vi "Finalize.vi"(8 "error in (no error)":errorcluster, 11 "Plugin in":refnum<class "Sift TDMS Uploader.lvclass">) -> (0 "error out":errorcluster, 3 "Plugin out":refnum<class "Sift TDMS Uploader.lvclass">)   [LabVIEW 2024, in "Sift TDMS Uploader.lvlib" / "Sift TDMS Uploader.lvclass"]
uses:
  Sift TDMS Uploader.lvclass
  Sift TDMS Uploader.lvclass/Sift TDMS Uploader.ctl
  <vilib>/FlexLogger/SDK/PluginSDK.lvlibp/PEFClasses/SDK/System Interface/System Interface.lvclass
  Globals.vi
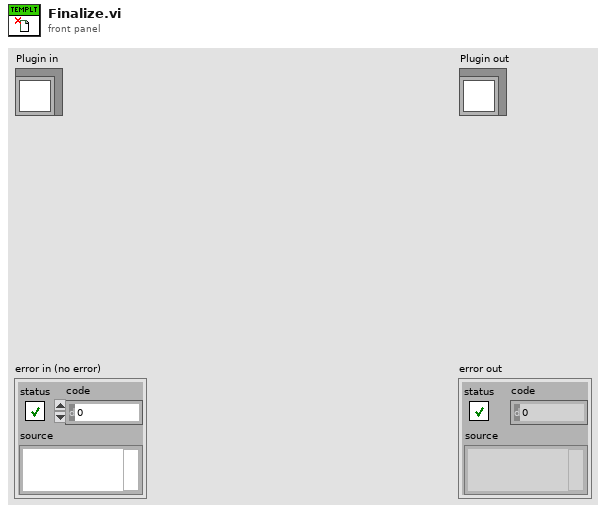
[diagram p1: front panel]
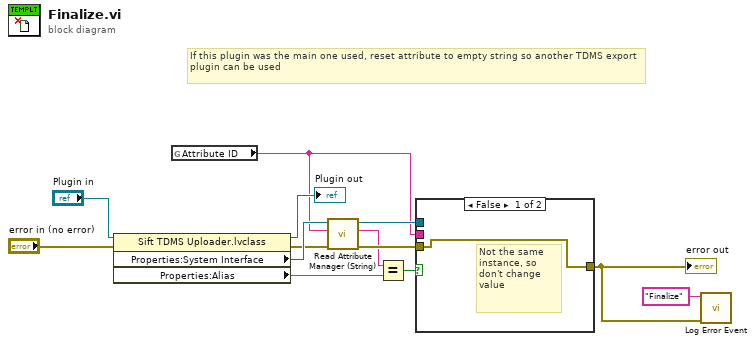
[diagram p0: block diagram]
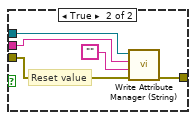
[diagram p2: hidden frame]
diagram:
  # "If this plugin was the main one used, reset attribute to empty string so another TDMS export plugin can be used"
  n1 = property class="Sift TDMS Uploader.lvclass"(reference="Plugin in", error in="error in (no error)") -> (reference out=→"Plugin out":refnum<class "Sift TDMS Uploader.lvclass">, error out=w12:errorcluster, "Properties:System Interface"=w13:refnum<class "System Interface.lvclass">, "Properties:Alias"=w8:string)
  n2 = global read "Globals.vi" "Attribute ID"() -> (w1:string)
  n3 = call-dynamic "Read Attribute Manager (String).vi"("error in (no error)"=w12, "Attribute ID"=w1, "System Interface in"=w13) -> ("error out"=w10:errorcluster, "Attrib Val"=w9:string, "System Interface out"=w11:refnum<class "System Interface.lvclass">)  [unwired: 5 in, 1 out]
  n4 = Equal?(x=w9, y=w8) -> (x = y?=w7:bool)
  n5 = case shown="False" w7 {
    tunnel: w11 -> [_ w19]
    tunnel: w10 -> [w14 w18]
    tunnel: w1 -> [_ w17]
    tunnel: [w14 w15] -> w2
    frame False {
      # "Not the same instance, so don't change value"
    }
    frame True {
      # "Reset value"
      n6 = call-dynamic "Write Attribute Manager (String).vi"("error in (no error)"=w18, "Attribute Value"="", "Attribute ID"=w17, "System Interface in"=w19) -> ("error out"=w15:errorcluster)  [unwired: 5 in, 2 out]
    }
  }
  "error out" <- w2
  n7 = call "Log Error Event.vi"("error in (no error)"=w2, "Location"="Finalize") -> ()  [unwired: 10 in]
